vi "Remove Target from Node Path.vi"(8 "error in (no error)":errorcluster, 11 "NodePath":string) -> (0 "error out":errorcluster, 3 "PathArrayToString":string)   [LabVIEW 2018, in "Instrument Addon System Explorer.lvlib"]
uses:
  Instrument Addon System Explorer.lvlib
  NationalInstruments.VeriStand
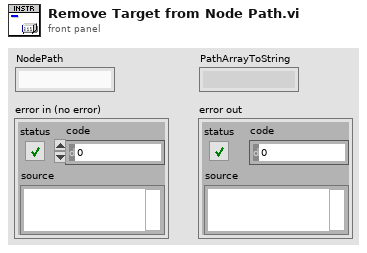
[diagram p1: front panel]
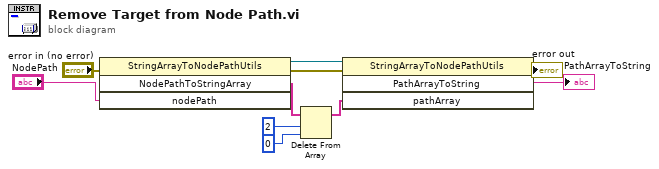
[diagram p0: block diagram]
diagram:
  n1 = invoke class="StringArrayToNodePathUtils" method="NodePathToStringArray"(error in="error in (no error)", "nodePath"="NodePath") -> (reference out=w10:refnum<k24>, error out=w7:errorcluster, "NodePathToStringArray"=w1:string[])  [unwired: 2 in, 1 out]
  n2 = Delete From Array(array=w1, length=2, index=0) -> (array with subset deleted=w6:string[])  [unwired: 1 out]
  n3 = invoke class="StringArrayToNodePathUtils" method="PathArrayToString"(reference=w10, error in=w7, "pathArray"=w6) -> (error out=→"error out":errorcluster, "PathArrayToString"=→"PathArrayToString":string)  [unwired: 1 in, 2 out]
